vi "Init Front Panel.vi"(7 "This VI":refnum<vi>, 8 "error in (no error)":errorcluster, 9 "Legend LB":refnum<vi>, 10 "Wfm Graph":refnum<vi>, 11 "Preview in":refnum<class "Preview.lvclass">) -> (0 "error out":errorcluster, 3 "Preview out":refnum<class "Preview.lvclass">)   [LabVIEW 2018, in "Preview Window.lvlib" / "Preview.lvclass"]
uses:
  Preview.lvclass
  <vilib>/Utility/miscctls.llb/LVRowAndColumnTypeDef.ctl
  Preview.lvclass/Preview.ctl
  Cfg Grandmaster/Class Chan Group/Read GroupChans.vi
  Cfg Grandmaster/Class Chan Group/Read GrpName.vi
  Cfg Grandmaster/Class Chan Group/Read MeasType.vi
  Measurements/Class Channel/Read ChanName.vi
  Measurements/Class Channel/Read Alias.vi
  Measurements/Class Channel/Channel.lvclass
  Cfg Grandmaster/Class Chassis Cfg/ChassisCfg.lvclass
  Cfg Grandmaster/Class Chan Group/ChanGrp.lvclass
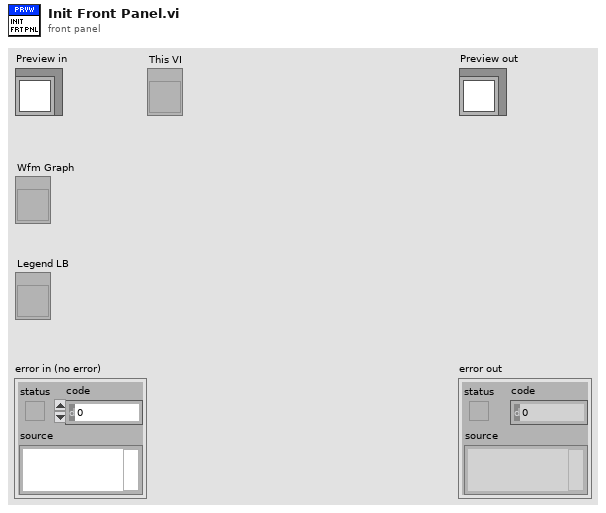
[diagram p1: front panel]
types:
  T1 = typedef "LVRowAndColumnTypeDef.ctl" = cluster{"Row":i32, "Column":i32}
  T2 = typedef "Selected Group.ctl" = cluster{"ChanGroup":i32, "Rate Class":T3}
  T3 = typedef "TE_Designator.ctl" = enum16{"High Speed", "Low Speed"}
  T4 = typedef "ge_MeasType.ctl" = enum16{"Voltage", "Frequency", "Tachometer", "Dynamic", "Thermocouple", "RTD", "Strain", "Current", "Resistance"}
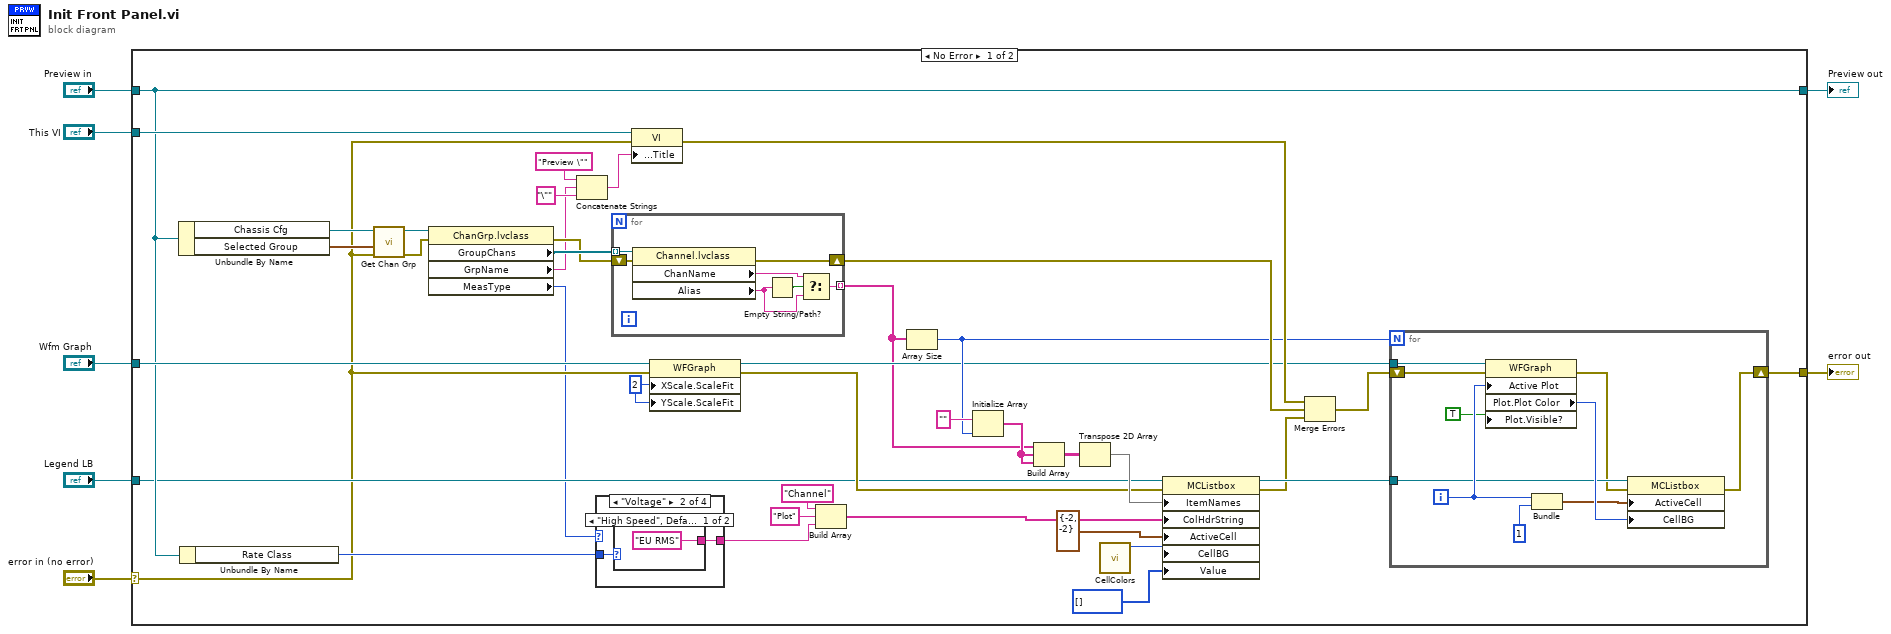
[diagram p0: block diagram]
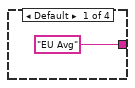
[diagram p2: hidden frame]
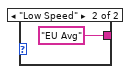
[diagram p3: hidden frame]
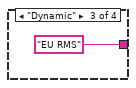
[diagram p4: hidden frame]
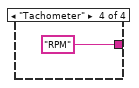
[diagram p5: hidden frame]
diagram:
  n1 = case shown="No Error" "error in (no error)" {
    selector: "error in (no error)" -> [w12 w72]
    tunnel: [w39 w72] -> w6
    tunnel: [w22 w71] -> w4
    tunnel: "Preview in" -> [w22 w71]
    tunnel: "This VI" -> [w38 _]
    tunnel: "Wfm Graph" -> [w24 _]
    tunnel: "Legend LB" -> [w19 _]
    frame No Error {
      w43 = u8 2 ("X Scale.Scale Fit")
      n2 = Unbundle By Name(w22) -> ("Chassis Cfg"=w37:refnum<class "ChassisCfg.lvclass">, "Selected Group"=w36:T2)
      n3 = Unbundle By Name(w22) -> ("Rate Class"=w23:T3)
      n4 = call "Get Chan Grp.vi"("error in (no error)"=w12, "Selected Grp"=w36, "Chassis Cfg"=w37) -> ("error out"=w34:errorcluster, "Chan Group"=w35:refnum<class "ChanGrp.lvclass">)  [unwired: 7 in]
      n5 = property class="ChanGrp.lvclass"(reference=w35, error in=w34) -> (error out=w32:errorcluster, "GroupChans"=w33:refnum<class "Channel.lvclass">[], "GrpName"=w10:string, "MeasType"=w11:T4)  [unwired: 1 out]
      n6 = Concatenate Strings("Preview \"", w10, "\"") -> (w26:string)
      n7 = case shown="\"Voltage\"" w11 {
        tunnel: ["EU Avg" w49 "EU RMS" "RPM"] -> w27
        tunnel: w23 -> [_ w48 _ _]
        frame Default {
        }
        frame "Voltage" {
          n8 = case shown="\"High Speed\", Default" w48 {
            tunnel: ["EU RMS" "EU Avg"] -> w49
            frame "High Speed", Default {
            }
            frame "Low Speed" {
            }
          }
        }
        frame "Dynamic" {
        }
        frame "Tachometer" {
        }
      }
      n9 = for {
        tunnel: [w59] -> w9 mode=indexing
        tunnel: w33 -> [w56] mode=indexing
        shift-right: [w54] -> w17
        shift-left: w32 -> [w55]
        n10 = property class="Channel.lvclass"(reference=w56, error in=w55) -> (error out=w54:errorcluster, "ChanName"=w57:string, "Alias"=w58:string)  [unwired: 1 out]
        n11 = Empty String/Path?(string/path=w58) -> (empty?=w60:bool)
        n12 = Select(t=w57, s=w60, f=w58) -> (s? t:f=w59:string)
      }
      n13 = property class="VI"(reference=w38, error in=w12, "Front Panel.Title"=w26) -> (error out=w18:errorcluster)  [unwired: 1 out]
      n14 = property on="Property Node" class="WFGraph"(reference=w24, error in=w12, "XScale.ScaleFit"=w43, "YScale.ScaleFit"=w43) -> (reference out=w13:refnum<vi>, error out=w21:errorcluster)
      n15 = Build Array("Channel", "Plot", w27) -> (w25:string[])
      n16 = Array Size(array=w9) -> (size(s)=w14:i32)
      n17 = Initialize Array("", w14) -> (w45:string[])
      n18 = Build Array(w9, w45, w45) -> (w44:string[][])
      n19 = Transpose 2D Array(2D array=w44) -> (transposed array=w40:string[][])
      n20 = call "CellColors.vi"() -> ("Normal"=w42:u32)  [unwired: 8 in, 3 out]
      n21 = property on="Property Node" class="MCListbox"(reference=w19, error in=w21, "ItemNames"=w40, "ColHdrString"=w25, "ActiveCell"=T1 {"Row"=-2, "Column"=-2} ("Active Cell:Active Cell"), "CellBG"=w42, "Value"=i32[] [] ("Legend LB")) -> (reference out=w20:refnum<vi>, error out=w16:errorcluster)
      n22 = Merge Errors(w18, w17, w16) -> (w15:errorcluster)
      n23 = for {
        N: w14 -> [_]
        shift-right: [w61] -> w39
        shift-left: w15 -> [w70]
        tunnel: w13 -> [w64]
        tunnel: w20 -> [w63]
        i -> [w68]
        n24 = property on="Property Node" class="WFGraph"(reference=w64, error in=w70, "Active Plot"=w68, "Plot.Visible?"=TRUE ("Plot.Visible")) -> (error out=w62:errorcluster, "Plot.Plot Color"=w69:u32)  [unwired: 1 out]
        n25 = Bundle(w68, 1) -> (w66:cluster{i32, i32})  [unwired: 1 in]
        n26 = property on="Property Node" class="MCListbox"(reference=w63, error in=w62, "ActiveCell"=w66, "CellBG"=w69) -> (error out=w61:errorcluster)  [unwired: 1 out]
      }
    }
    frame Error {
    }
  }
  "error out" <- w6
  "Preview out" <- w4
